vi "file.open.vi"(8 "error in":errorcluster, 11 "Path to MIDI File (use dialog)":path) -> (0 "error out":errorcluster, 3 "midi-file out":refnum<class "midi-file.lvclass">)   [LabVIEW 2020, in "midi-file.lvclass"]
uses:
  midi-file.lvclass
  midi-file.lvclass/midi-file.ctl
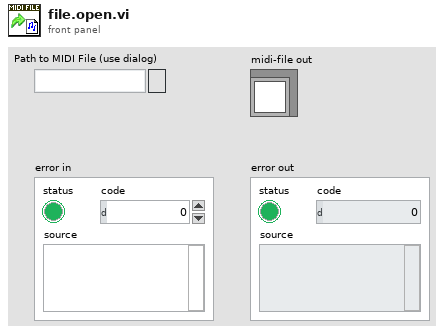
[diagram p1: front panel]
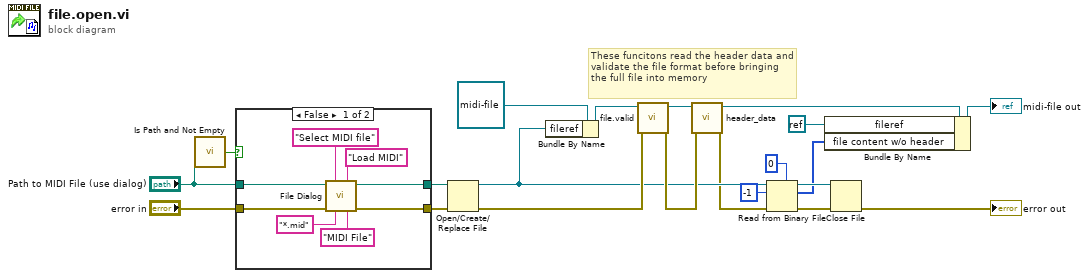
[diagram p0: block diagram]
diagram:
  # "These funcitons read the header data and validate the file format before bringing the full file into memory"
  n1 = call <vilib>:"Is Path and Not Empty.vi"("path"="Path to MIDI File (use dialog)") -> ("Is Path and Not Empty?"=w5:bool)  [unwired: 4 in]
  n2 = case shown="False" w5 {
    tunnel: [w24 w31] -> w4
    tunnel: "error in" -> [w23 w31]
    tunnel: "Path to MIDI File (use dialog)" -> [w26 w30]
    tunnel: [w25 w30] -> w1
    frame False {
      n3 = call "File Dialog"("start path"=w26, "prompt"="Select MIDI file", "button label"="Load MIDI", "error in"=w23, "pattern (all files)"="*.mid", "pattern label"="MIDI File") -> ("selected path"=w25:path, "error out"=w24:errorcluster)  [unwired: 6 in, 2 out]
    }
    frame True {
    }
  }
  n4 = Open/Create/Replace File(file path (use dialog)=w1, error in=w4) -> (refnum out=w16:refnum<file>, error out=w19:errorcluster)  [unwired: 4 in, 1 out]
  n5 = Bundle By Name(cluster=refnum<class "midi-file.lvclass"> refnum ("midi-file out"), "fileref"=w16) -> (w20:refnum<class "midi-file.lvclass">)
  n6 = call "file.valid.vi"("error in"=w19, "midi-file in"=w20) -> ("error out"=w17:errorcluster, "midi-file out"=w18:refnum<class "midi-file.lvclass">)  [unwired: 8 in]
  n7 = call "header_data.vi"("error in"=w17, "midi-file in"=w18) -> ("error out"=w11:errorcluster, "midi-file out"=w9:refnum<class "midi-file.lvclass">)  [unwired: 8 in]
  n8 = Read from Binary File(5:u8 0, 8:w11, 10:-1 ("count (1)"), 11:w16) -> (0:w12:errorcluster, 2:w7:u8[], 3:w13:refnum<file>)  [unwired: 2 in, 1 out]
  n9 = Bundle By Name(cluster=w9, "fileref"=refnum<k0> refnum, "file content w/o header"=w7) -> (→"midi-file out":refnum<class "midi-file.lvclass">)
  n10 = Close File(refnum=w13, error in=w12) -> (error out=→"error out":errorcluster)  [unwired: 1 out]
